vi "XY Graph Load Plot(s) Event.vi"(7 "Max Number of Plot to Load (-1: All)":i32=-1, 8 "Error In":errorcluster, 11 "XYGraph Ref":refnum<vi>) -> (0 "Error Out":errorcluster, 1 "Message":string, 2 "File Path(s)":path[](array[path]), 3 "Loaded Plot Names":cluster{"Plot Names":string[]}[](array[cluster]), 4 "# Plots Added":i32[](array[numeric]), 5 "Graph Caption (or Label)":string)   [LabVIEW 2019, in "XY Graph Add-Ons.lvlib"]
uses:
  XY Graph Add-Ons.lvlib
  ASCII File Header Definition.ctl
  <vilib>/Utility/error.llb/Error Cluster From Error Code.vi
  <vilib>/ErrorRing/Error Ring.xnode
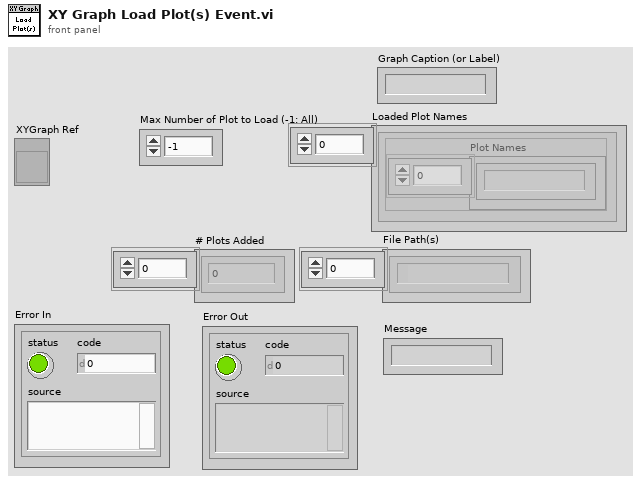
[diagram p1: front panel]
types:
  T1 = typedef "XY Graph Add-Ons.lvlib/XY Graph Refnum.ctl" = refnum<vi>
  T2 = typedef "ASCII File Header Definition.ctl" = cluster{"Number of Lines to Skip":i32, "Column Header Line?":bool}
  T3 = typedef "Plot Scale Labels.ctl" = cluster{"X Scale Label":string, "Y Scale Label":string}
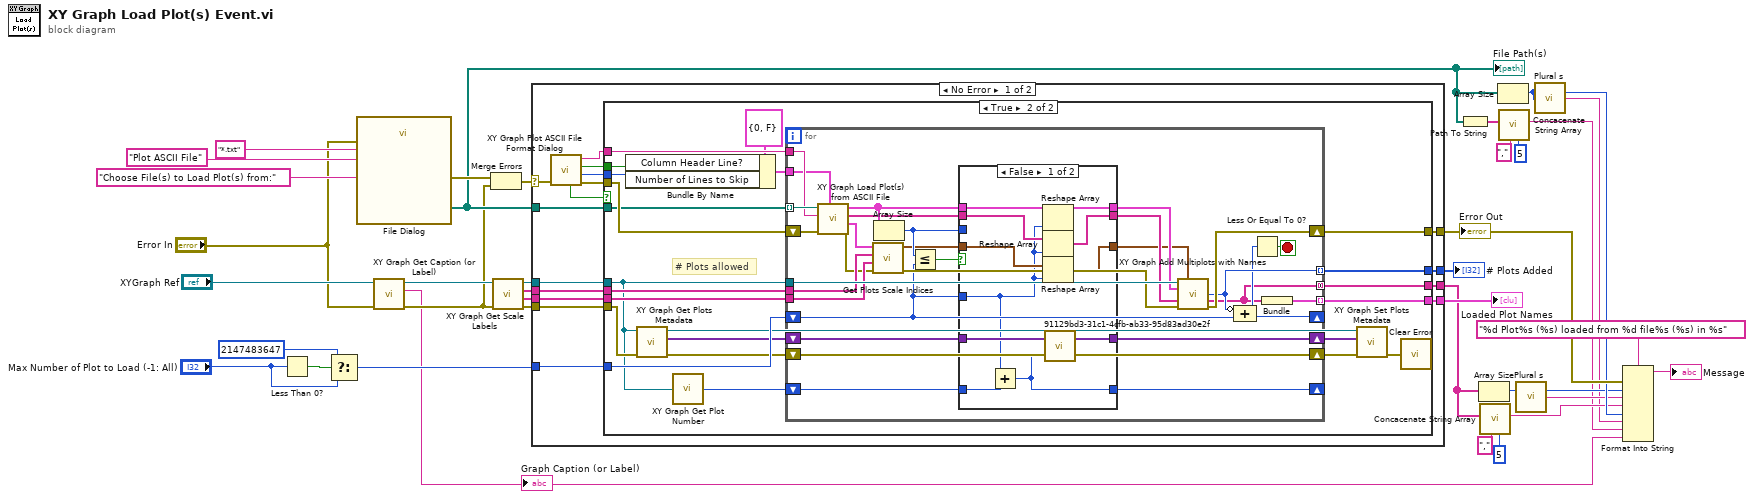
[diagram p0: block diagram]
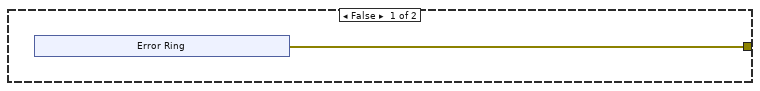
[diagram p2: hidden frame]
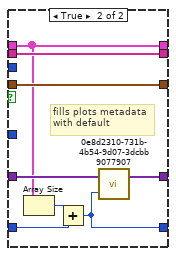
[diagram p3: hidden frame]
diagram:
  n1 = Less Than 0?(x="Max Number of Plot to Load (-1: All)") -> (x < 0?=w24:bool)
  n2 = Select(t=2147483647 ("Max Number of Plot to Load (-1: All)"), s=w24, f="Max Number of Plot to Load (-1: All)") -> (s? t:f=w21:i32)
  n3 = call "File Dialog"("prompt"="Choose File(s) to Load Plot(s) from:", "error in"="Error In", "pattern (all files)"="*.txt", "pattern label"="Plot ASCII File") -> ("selected paths"=w13:path[], "error out"=w31:errorcluster)  [unwired: 8 in, 2 out]
  "File Path(s)" <- w13
  n4 = call "XY Graph Get Caption (or Label).vi"("error in (no error)"="Error In", "XYGraph in"="XYGraph Ref") -> ("error out"=w3:errorcluster, "Caption (or Label) Text"=w2:string, "XYGraph out"=w35:T1)  [unwired: 7 in]
  "Graph Caption (or Label)" <- w2
  n5 = Merge Errors(w31, w3) -> (w30:errorcluster)
  n6 = call "XY Graph Get Scale Labels.vi"("Error In"=w3, "XYGraph in"=w35) -> ("Error Out"=w1:errorcluster, "Y Scale Labels"=w27:string[], "X Scale Labels"=w28:string[], "XYGraph out"=w29:T1)  [unwired: 4 in, 2 out]
  n7 = case shown="No Error" w30 {
    selector: w30 -> [w52 w130]
    tunnel: w29 -> [w45 _]
    tunnel: w13 -> [w46 _]
    tunnel: [w44 _] -> w26
    tunnel: w28 -> [w43 _]
    tunnel: w27 -> [w42 _]
    tunnel: [w41 w130] -> w12
    tunnel: [w40 _] -> w25
    tunnel: w21 -> [w39 _]
    tunnel: [w38 _] -> w20
    tunnel: w1 -> [w37 _]
    frame No Error {
      n8 = call "XY Graph Plot ASCII File Format Dialog.vi"("error in (no error)"=w52) -> ("error out"=w50:errorcluster, "Number of Lines to Skip"=w47:i32, "Column Header Line?"=w48:bool, "Separator"=w49:string, "OK"=w51:bool)  [unwired: 6 in]
      n9 = case shown="True" w51 {
        tunnel: w50 -> [_ w80]
        tunnel: w49 -> [_ w77]
        tunnel: w48 -> [_ w76]
        tunnel: w47 -> [_ w75]
        tunnel: w46 -> [_ w78]
        tunnel: w45 -> [_ w63]
        tunnel: [_ w79] -> w44
        tunnel: w43 -> [_ w72]
        tunnel: w42 -> [_ w71]
        tunnel: [w53 w70] -> w41
        tunnel: [_ w69] -> w40
        tunnel: w39 -> [_ w68]
        tunnel: [_ w67] -> w38
        tunnel: w37 -> [_ w66]
        frame False {
          n10 = xnode "Error Ring"() -> ("error out"=w53:errorcluster)
        }
        frame True {
          # "# Plots allowed"
          n11 = Bundle By Name(cluster=T2 {"Number of Lines to Skip"=0, "Column Header Line?"=FALSE} ("Header Definitions"), "Column Header Line?"=w76, "Number of Lines to Skip"=w75) -> (w73:T2)
          n12 = call "XY Graph Get Plots Metadata.vi"("Error In"=w66, "XYGraph Refnum"=w63) -> ("Error Out"=w65:errorcluster, "Plots Metadata"=w64:variant[], "XYGraph Refnum"=w59:T1)  [unwired: 6 in, 1 out]
          n13 = call "XY Graph Get Plot Number.vi"("XYGraph"=w63) -> ("# Plots"=w62:i32)  [unwired: 8 in]
          n14 = for {
            tunnel: w63 -> [w110]
            tunnel: [w100] -> w79 mode=indexing
            tunnel: w78 -> [w109] mode=indexing
            tunnel: w77 -> [w107]
            tunnel: w73 -> [w106]
            tunnel: w72 -> [w105]
            tunnel: w71 -> [w104]
            shift-right: [w99] -> w70
            shift-left: w80 -> [w108]
            tunnel: [w93] -> w69 mode=indexing
            shift-right: [w92] -> _
            shift-left: w68 -> [w87]
            tunnel: [w86] -> w67 mode=concatenating
            shift-right: [w82] -> w61
            shift-left: w65 -> [w82]
            shift-right: [w83] -> w58
            shift-left: w64 -> [w85]
            shift-right: [w81] -> _
            shift-left: w62 -> [w84]
            stop <- w91 stop-if-true
            n15 = call "XY Graph Load Plot(s) from ASCII File.vi"("Header Definitions"=w106, "error in (no error)"=w108, "Delimiter (TAB)"=w107, "File Path"=w109) -> ("error out"=w102:errorcluster, "Plot Scales Array"=w103:T3[], "Plot Name Array"=w95:string[], "Plot Array"=w96:cluster{"X Array":dbl[], "Y Array":dbl[]}[])  [unwired: 4 in]
            n16 = call "Get Plots Scale Indices.vi"("Error In"=w102, "Y Scale Labels"=w104, "X Scale Labels"=w105, "Plot Scales Array"=w103) -> ("Error Out"=w101:errorcluster, "Array of Scales (Default)"=w94:cluster{"X Scale":u32, "Y Scale":u32}[])  [unwired: 6 in]
            n17 = Array Size(array=w96) -> (size(s)=w97:i32)
            n18 = Less Or Equal?(x=w97, y=w87) -> (x <= y?=w98:bool)
            n19 = case shown="False" w98 {
              tunnel: w97 -> [_ _]
              tunnel: w96 -> [w121 w126]
              tunnel: w95 -> [w117 w129]
              tunnel: w94 -> [w119 w128]
              tunnel: [w120 w126] -> w90
              tunnel: [w116 w129] -> w89
              tunnel: [w118 w128] -> w88
              tunnel: w87 -> [w112 _]
              tunnel: w85 -> [w115 w127]
              tunnel: w84 -> [w113 w124]
              tunnel: [w114 w123] -> w83
              tunnel: [w111 w122] -> w81
              frame False {
                n20 = Add(x=w112, y=w113) -> (x+y=w111:i32)
                n21 = Reshape Array(w121, w112) -> (w120:cluster{"X Array":dbl[], "Y Array":dbl[]}[])
                n22 = Reshape Array(w117, w112) -> (w116:string[])
                n23 = Reshape Array(w119, w112) -> (w118:cluster{"X Scale":u32, "Y Scale":u32}[])
                n24 = call "91129bd3-31c1-4cfb-ab33-95d83ad30e2f.vi"("dimension size"=w111, "1D Array"=w115) -> ("1D Array"=w114:variant[])  [unwired: 1 in]
              }
              frame True {
                # "fills plots metadata\nwith default"
                n25 = Array Size(array=w126) -> (size(s)=w125:i32)
                n26 = Add(x=w125, y=w124) -> (x+y=w122:i32)
                n27 = call "0e8d2310-731b-4b54-9d07-3dcbb9077907.vi"("dimension size"=w122, "1D Array"=w127) -> ("1D Array"=w123:variant[])  [unwired: 1 in]
              }
            }
            n28 = call "XY Graph Add Multiplots with Names.vi"("XYGraph in"=w110, "Array of Scales (Default)"=w88, "Array of Plots"=w90, "Array of Plot Names (\"Plot\")"=w89, "error in (no error)"=w101) -> ("Number of Plots Added"=w93:i32, "Added Plot Names"=w86:string[], "error out"=w99:errorcluster)  [unwired: 6 in, 2 out]
            n29 = Compound Arithmetic op=ADD(invert w93, w87) -> (w92:i32)
            n30 = Less Or Equal To 0?(x=w92) -> (x <= 0?=w91:bool)
            n31 = Bundle("Added Plot Names"=w86) -> (w100:cluster{"Added Plot Names":string[]})  [unwired: 1 in]
          }
          n32 = call "XY Graph Set Plots Metadata.vi"("error in (no error)"=w61, "Plots Metadata"=w58, "XY Graph Refnum"=w59) -> ("error out"=w60:errorcluster)  [unwired: 7 in, 1 out]
          n33 = call "Clear Error.vi"("Error In"=w60) -> ()  [unwired: 8 in, 1 out]
        }
      }
    }
    frame Error {
    }
  }
  "Error Out" <- w12
  "Loaded Plot Names" <- w26
  "# Plots Added" <- w25
  n34 = Path To String(path=w13) -> (string=w14:string[])
  n35 = Array Size(array=w20) -> (size(s)=w9:i32)
  n36 = call "Concacenate String Array.vi"("Max Number of Elements (None: -1)"=5 ("Max Number of Elements (None: 1)"), "Separator (TAB)"=",", "String Array"=w20) -> ("Formatted String"=w7:string)  [unwired: 8 in]
  n37 = Array Size(array=w13) -> (size(s)=w10:i32)
  n38 = call "Concacenate String Array.vi"("Max Number of Elements (None: -1)"=5 ("Max Number of Elements (None: 1)"), "Separator (TAB)"=",", "String Array"=w14) -> ("Formatted String"=w6:string)  [unwired: 8 in]
  n39 = call "Plural s.vi"("# Elements"=w9) -> ("Plural s"=w8:string)
  n40 = call "Plural s.vi"("# Elements"=w10) -> ("Plural s"=w5:string)
  n41 = Format Into String(format string="%d Plot%s (%s) loaded from %d file%s (%s) in %s", error in=w12, w9, w8, w7, w10, w5, w6, w2) -> (resulting string=→"Message":string)  [unwired: 1 in, 1 out]
